vi "Select_Value.vi"(3 "Numerisch":i32, 5 "System Monitor Variables":T1) -> (0 "Array":dbl[](array[numeric]), 1 "String":string, 2 "Value":dbl format="%#_13g")   [LabVIEW 2019]
uses:
  Global/Global Variables/System Monitor Cluster.ctl
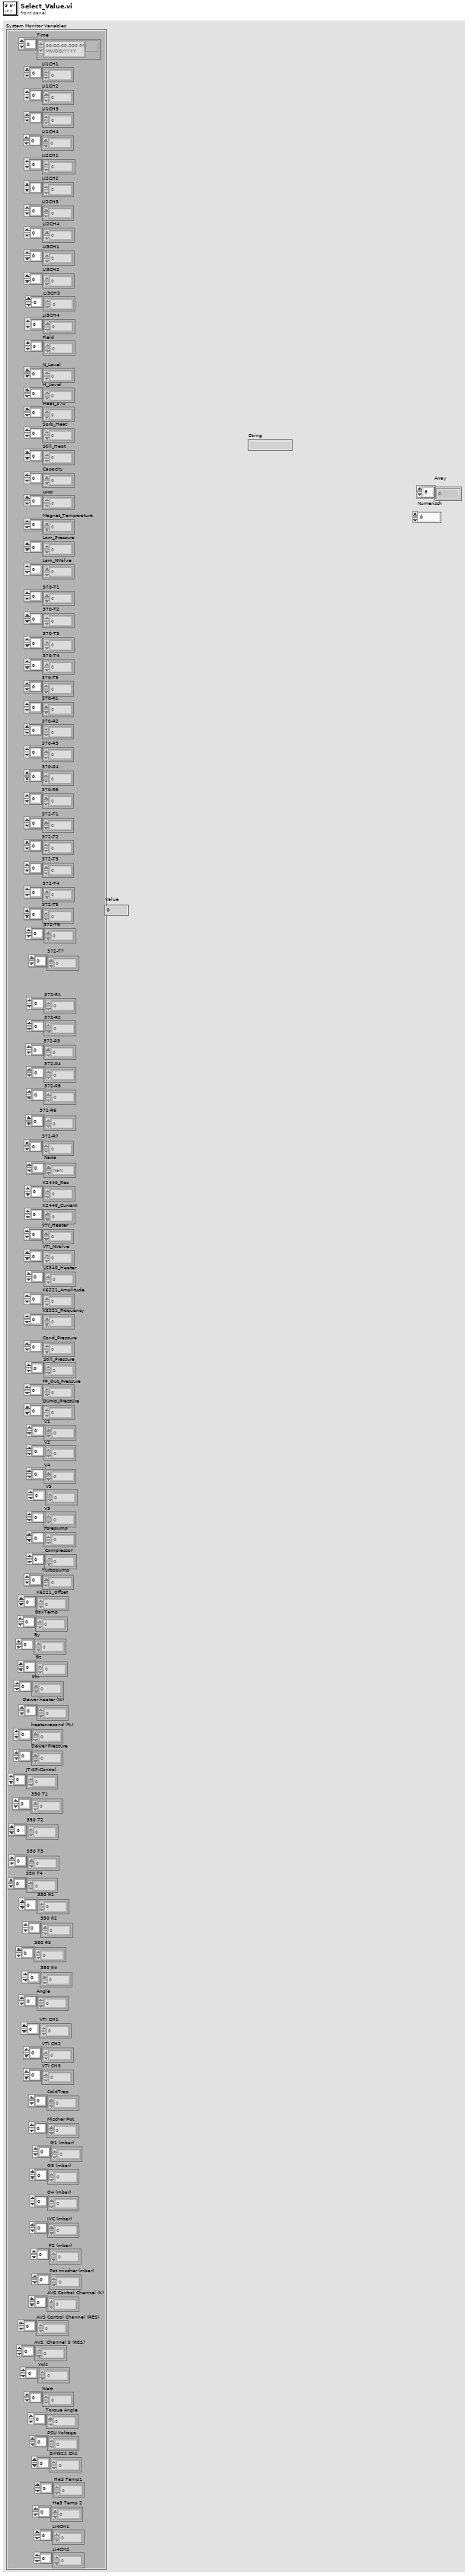
[diagram p1: front panel]
types:
  T1 = typedef "System Monitor Cluster.ctl" = cluster{"Time":timestamp[], "LI1CH1":dbl[], "LI1CH2":dbl[], "LI2CH1":dbl[], "LI2CH2":dbl[], "LI3CH1":dbl[], "LI3CH2":dbl[], "Field":dbl[], "N_Level":dbl[], "H_Level":dbl[], "Heat_370":dbl[], "Sorb_Heat":dbl[], "Still_Heat":dbl[], "Capacity":dbl[], "Loss":dbl[], "Magnet_Temperature":dbl[], "Lam_Pressure":dbl[], "Lam_NValve":dbl[], "370-T1":dbl[], "370-T2":dbl[], "370-T3":dbl[], "370-T4":dbl[], "370-T5":dbl[], "370-R1":dbl[], "370-R2":dbl[], "370-R3":dbl[], "370-R4":dbl[], "370-R5":dbl[], "372-T1":dbl[], "372-T2":dbl[], "372-T3":dbl[], "372-T4":dbl[], "372-T5":dbl[], "372-T6":dbl[], "372-R1":dbl[], "372-R2":dbl[], "372-R3":dbl[], "372-R4":dbl[], "372-R5":dbl[], "372-R6":dbl[], "Nada":dbl[], "K2440_Res":dbl[], "K2440_Current":dbl[], "VTI_Heater":dbl[], "VTI_NValve":dbl[], "LS340_Heater":dbl[], "K6221_Amplitude":dbl[], "K6221_Frequency":dbl[], "Cond_Pressure":dbl[], "Still_Pressure":dbl[], "FP_Out_Pressure":dbl[], "Dump_Pressure":dbl[], "V1":dbl[], "V2":dbl[], "V4":dbl[], "V5":dbl[], "V9":dbl[], "Forepump":dbl[], "Compressor":dbl[], "K6221_Offset":dbl[], "BoxTemp":dbl[], "By":dbl[], "Bz":dbl[], "Phi":dbl[], "heater-recond (%)":dbl[], "Dewar Pressure ":dbl[], "JT-SP-Control":dbl[], "350 T1":dbl[], "350 T2":dbl[], "350 T3":dbl[], "350 T4":dbl[], "350 R1":dbl[], "350 R2":dbl[], "350 R3":dbl[], "350 R4":dbl[], "Angle":dbl[], "VTI CH1":dbl[], "VTI CH2":dbl[], "VTI CH3":dbl[], "ColdTrap":dbl[], "Mischer Pot":dbl[], "G1 (mbar)":dbl[], "G3 (mbar) ":dbl[], "G4 (mbar)":dbl[], "IVC (mbar)":dbl[], "P2 (mbar) ":dbl[], "Pot mischer (mbar)":dbl[], "AVS Control Channel (K)":dbl[], "AVS Control Channel (RES)":dbl[], "AVS  Channel 5 (RES) ":dbl[], "LI3CH3":dbl[], "LI3CH4":dbl[], "LI1CH3":dbl[], "LI1CH4":dbl[], "LI2CH3":dbl[], "LI2CH4":dbl[], "Volt":dbl[], "Watt":dbl[], "Torque Angle":dbl[], "Dewar heater (W)":dbl[], "PSU Voltage":dbl[], "Turbopump":dbl[], "372-R7":dbl[], "372-T7":dbl[], "SIM921 Ch1":dbl[], " He3 Temp1":dbl[], " He3 Temp 2":dbl[], "LI4CH1":dbl[], "LI4CH2":dbl[]}
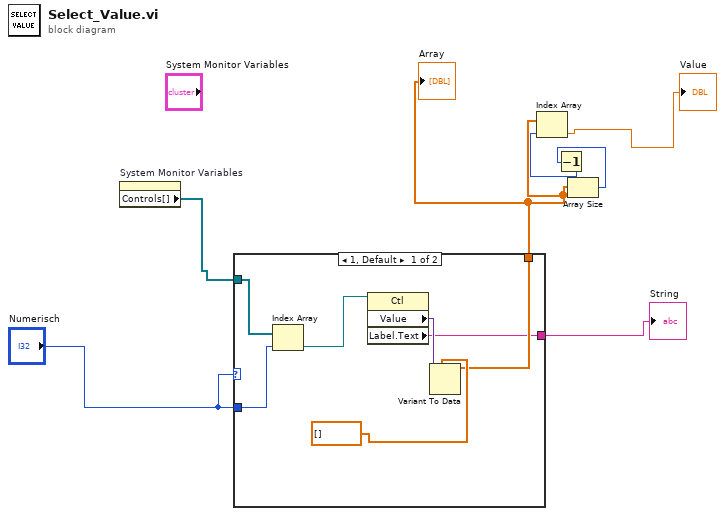
[diagram p0: block diagram]
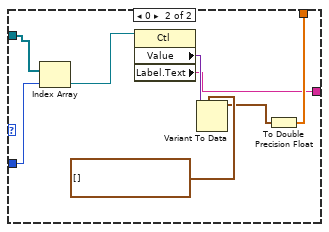
[diagram p2: hidden frame]
diagram:
  n1 = property on="System Monitor Variables" class="Clust (strict)"() -> ("Controls[]"=w7:refnum<vi>[])  [unwired: 2 in, 2 out]
  n2 = case shown="1, Default" "Numerisch" {
    tunnel: w7 -> [w12 w22]
    tunnel: "Numerisch" -> [w11 w20]
    tunnel: [w9 w17] -> w3
    tunnel: [w8 w16] -> w1
    frame 1, Default {
      n3 = Index Array(array=w12, index=w11) -> (element=w13:refnum<vi>)
      n4 = property class="Ctl"(reference=w13) -> ("Value"=w14:variant, "Label.Text"=w8:string)  [unwired: 1 in, 2 out]
      n5 = Variant To Data(type=dbl[] [] ("Array 3"), Variant=w14) -> (data=w9:dbl[])  [unwired: 1 in, 1 out]
    }
    frame 0 {
      n6 = Index Array(array=w22, index=w20) -> (element=w21:refnum<vi>)
      n7 = property class="Ctl"(reference=w21) -> ("Value"=w19:variant, "Label.Text"=w16:string)  [unwired: 1 in, 2 out]
      n8 = Variant To Data(type=timestamp[] [] ("Time"), Variant=w19) -> (data=w15:timestamp[])  [unwired: 1 in, 1 out]
      n9 = To Double Precision Float(number=w15) -> (double precision float=w17:dbl[])
    }
  }
  "Array" <- w3
  "String" <- w1
  n10 = Array Size(array=w3) -> (size(s)=w6:i32)
  n11 = Decrement(x=w6) -> (x-1=w5:i32)
  n12 = Index Array(array=w3, index=w5) -> (element=→"Value":dbl)
